vi "Off.vi"(8 "error in (no error)":errorcluster, 11 "Quartz in":refnum<class "Quartz.lvclass">) -> (0 "error out":errorcluster, 3 "Quartz out":refnum<class "Quartz.lvclass">)   [LabVIEW 2016, in "Quartz.lvclass"]
uses:
  Quartz.lvclass
  LightBox/LightBox.lvclass
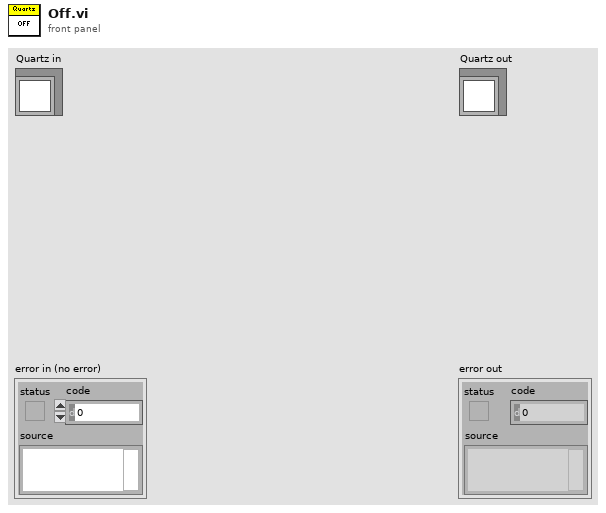
[diagram p1: front panel]
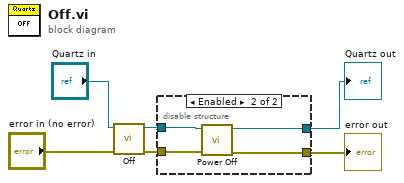
[diagram p0: block diagram]
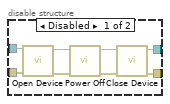
[diagram p2: hidden frame]
diagram:
  n1 = call-parent "Off.vi"("error in (no error)"="error in (no error)", "Lamp in"="Quartz in") -> ("error out"=w3:errorcluster, "Lamp out"=w4:refnum<class "Quartz.lvclass">)  [unwired: 8 in]
  n2 = disable-structure shown="Enabled" {
    disable-tunnel: w4 -> [w14 w18]
    disable-tunnel: w3 -> [w13 w16]
    disable-tunnel: [w10 w15] -> w2
    disable-tunnel: [w7 w17] -> w1
    frame Disabled {
      n3 = call-dynamic "Open Device.vi"("error in (no error)"=w13, "LightBox in"=w14) -> ("error out"=w12:errorcluster, "LightBox out"=w9:refnum<class "Quartz.lvclass">)  [unwired: 8 in]
      n4 = call-dynamic "Power Off.vi"("error in (no error)"=w12, "Quartz in"=w9) -> ("error out"=w11:errorcluster, "Quartz out"=w8:refnum<class "Quartz.lvclass">)  [unwired: 8 in]
      n5 = call-dynamic "Close Device.vi"("error in (no error)"=w11, "LightBox in"=w8) -> ("error out"=w10:errorcluster, "LightBox out"=w7:refnum<class "Quartz.lvclass">)  [unwired: 8 in]
    }
    frame Enabled {
      n6 = call-dynamic "Power Off.vi"("error in (no error)"=w16, "Quartz in"=w18) -> ("error out"=w15:errorcluster, "Quartz out"=w17:refnum<class "Quartz.lvclass">)  [unwired: 8 in]
    }
  }
  "error out" <- w2
  "Quartz out" <- w1
